vi "MeasureRMS.vi"(10 "Sample number":i32=100, 11 "Sample Rate (hz)":dbl=1000.0) -> (2 "Waveform Graph":dynamicdata(graph), 3 "RMS":dbl)   [LabVIEW 2015]
uses:
  <vilib>/Analysis/5stat.llb/RMS (DBL).vi
  <vilib>/Analysis/NI_AALPro.lvlib
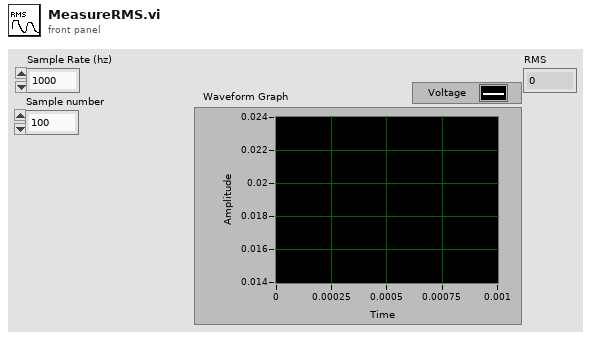
[diagram p1: front panel]
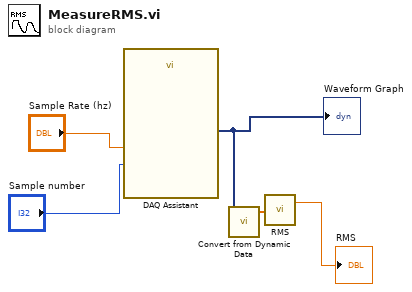
[diagram p0: block diagram]
diagram:
  n1 = call "DAQ Assistant"("rate"="Sample Rate (hz)", "number of samples"="Sample number") -> ("data"=w3:dynamicdata)  [unwired: 15 in, 2 out]
  "Waveform Graph" <- w3
  n2 = call "Convert from Dynamic Data"("Dynamic Data Type"=w3) -> ("Array"=w2:dbl[])  [unwired: 3 in]
  n3 = call-poly <vilib>:"RMS.vi"("X"=w2) -> ("rms value"=→"RMS":dbl)  [unwired: 1 out]
